vi "Destructor.vi"(8 "error in (no error)":errorcluster, 11 "Keithley 2400 in":refnum<class "Keithley 2400.lvclass">) -> (0 "error out":errorcluster, 3 "Keithley 2400 out":refnum<class "Keithley 2400.lvclass">)   [LabVIEW 2011, in "Keithley 2400.lvclass"]
uses:
  Keithley 2400.lvclass
  Keithley 2400.lvclass/Keithley 2400.ctl
  <instrlib>/Keithley 24XX/Keithley 24XX.lvlib
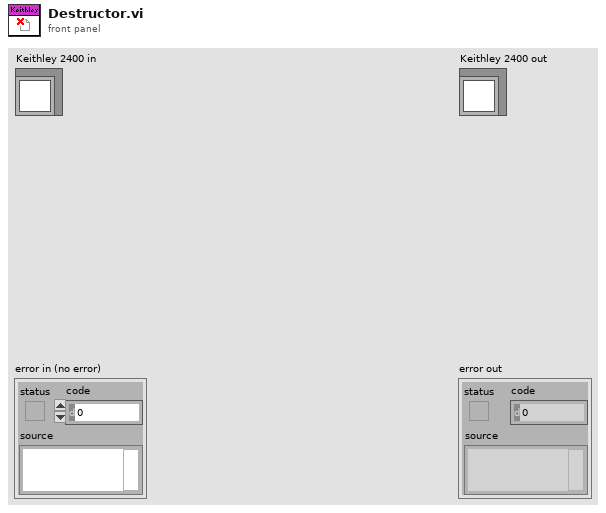
[diagram p1: front panel]
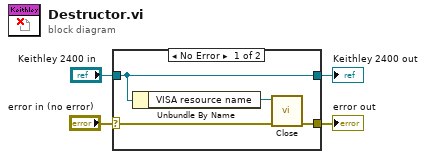
[diagram p0: block diagram]
diagram:
  n1 = case shown="No Error" "error in (no error)" {
    selector: "error in (no error)" -> [w6 w10]
    tunnel: [w5 w10] -> w3
    tunnel: [w7 w9] -> w1
    tunnel: "Keithley 2400 in" -> [w7 w9]
    frame No Error {
      n2 = Unbundle By Name(w7) -> ("VISA resource name"=w8:refnum<visa-resource-name>)
      n3 = call <instrlib>:"Close.vi"("error in (no error)"=w6, "VISA resource name"=w8) -> ("error out"=w5:errorcluster)  [unwired: 9 in]
    }
    frame Error {
    }
  }
  "error out" <- w3
  "Keithley 2400 out" <- w1
